vi "LINX - MMA8452Q Accelerometer.vi"() -> ()   [LabVIEW 2019]
doc: "This example demonstrates how to read X, Y, and Z accelerations using the MMA8452 accelerometer."
uses:
  <vilib>/MakerHub/LINX/Public/Utilities/Open Serial.vi
  <vilib>/MakerHub/LINX/LMH-LINX.lvlib
  <vilib>/MakerHub/LINX/Public/Sensors/Accelerometer/MMA8452/MMA8452.lvlib
panel:
  in  "Stop Button":bool
  out "Waveform Chart":T1(graph)
  in  "I2C Channel":u8
  in  "Serial Port":refnum<visa-resource-name>
  out "Loop Rate (Hz)":u32
  # "MMA8452Q Accelerometer\n\nThis example demonstrates how to read three axis of acceleration from the MMA8452Q accelerometer \n\nInstructions\n1. Select the COM Port associated with the LINX Device.\n2. Select the I2C Channel that the MMA8452Q is connected to.\n3. Click the Run Arrow."
  # "LINX Device Settings"
  # "Analog Value"
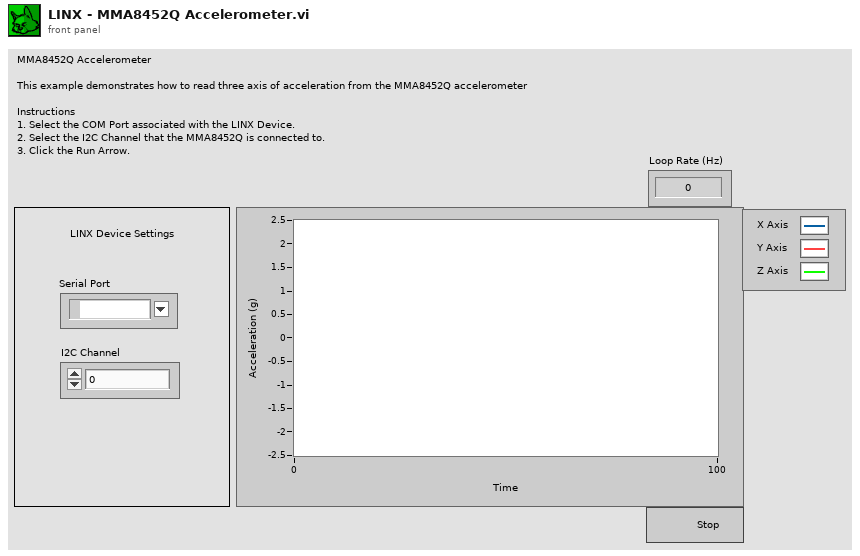
[diagram p1: front panel]
types:
  T1 = cluster{"X Axis":dbl, "Y Axis":dbl, "Z Axis":dbl}
  T2 = typedef "LMH-LINX.lvlib/LINX Ref.ctl" = cluster{"IO":T3, "Interface":T4, "LINX Device Config":T5}
  T3 = typedef "LMH-LINX.lvlib/Platform.ctl" = enum16{"Remote", "Local"}
  T4 = typedef "LMH-LINX.lvlib/Interface.ctl" = enum16{"Serial", "TCP"}
  T5 = typedef "LMH-LINX.lvlib/Device.lvlib/LINX Device Config.ctl" = cluster{"Interface":T4, "COM Port":refnum<visa-resource-name>, "TCP Configuration":T6, "Device Family":u8, "Device ID":u8, "Device Name":string, "TCP Ref":refnum<k5>, "Channels":T7}
  T6 = typedef "LMH-LINX.lvlib/Device.lvlib/TCP Config.ctl" = cluster{"IP Address":string, "Port":u16}
  T7 = typedef "LMH-LINX.lvlib/Channels.ctl" = cluster{"DI":u8[], "DO":u8[], "AI":u8[], "AO":u8[], "PWM":u8[], "QE":u8[], "UART":u8[], "I2C 2":u8[], "SPI":u8[], "CAN":u8[], "Servo":u8[], "AI Ref (V)":dbl, "AI Resolution (Bits)":u8, "AO Ref (V)":dbl, "AO Resolution (Bits)":u8}
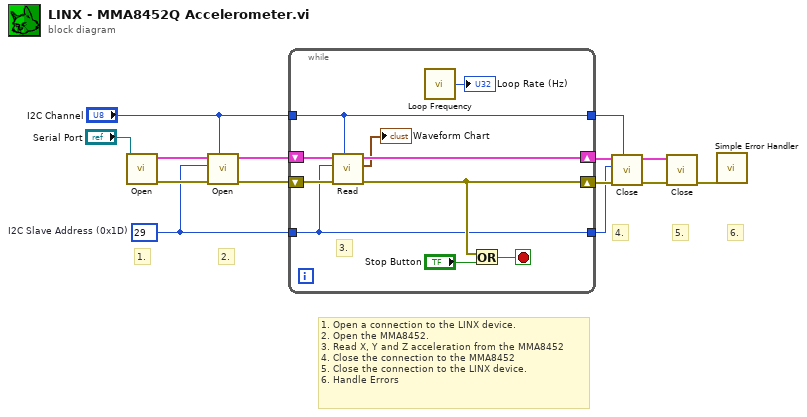
[diagram p0: block diagram]
diagram:
  w8 = u8 29  # I2C Slave Address (0x1D)
  # "6."
  # "4."
  # "2."
  # "5."
  # "1. Open a connection to the LINX device.\n2. Open the MMA8452.\n3. Read X, Y and Z acceleration from the MMA8452\n4. Close the connection to the MMA8452\n5. Close the connection to the LINX device.\n6. Handle Errors"
  # "1."
  n1 = call-poly <vilib>:"Open.vi"("Serial Port"="Serial Port") -> ("Error Out"=w13:errorcluster, "LINX Resource"=w12:T2)  [unwired: 8 in, 1 out]
  n2 = call <vilib>:"Open.vi"("I2C Channel"="I2C Channel", "Error In"=w13, "I2C Slave Address (0x1D)"=w8, "LINX Ref"=w12) -> ("Error Out"=w10:errorcluster, "LINX Resource"=w11:T2)  [unwired: 6 in]
  n3 = while {
    tunnel: "I2C Channel" -> [w17]
    tunnel: w8 -> [w15]
    shift-right: [w20] -> w5
    shift-left: w11 -> [w19]
    shift-right: [w22] -> w6
    shift-left: w10 -> [w24]
    tunnel: [w17] -> w2
    tunnel: [w15] -> w1
    stop <- w21 stop-if-true
    # "3."
    n4 = call <vilib>:"Read.vi"("I2C Channel"=w17, "Error In"=w24, "I2C Slave Address (0x1D)"=w15, "LINX Resource in"=w19) -> ("Error Out"=w22:errorcluster, "Acceleration Data (g)"=→"Waveform Chart":T1, "LINX Resource out"=w20:T2)  [unwired: 5 in]
    n5 = call <vilib>:"Loop Frequency.vi"() -> ("Loop Rate (Hz)"=→"Loop Rate (Hz)":u32)
    n6 = Or(x=w22, y="Stop Button") -> (x .or. y?=w21:bool)
  }
  n7 = call <vilib>:"Close.vi"("I2C Channel (0)"=w2, "Error In"=w6, "I2C Slave Address (0)"=w1, "LINX Resource"=w5) -> ("Error Out"=w3:errorcluster, "LINX Resource"=w4:T2)  [unwired: 6 in]
  n8 = call <vilib>:"Close.vi"("Error In"=w3, "LINX Resource"=w4) -> ("Error Out"=w7:errorcluster)  [unwired: 9 in]
  n9 = call <vilib>:"Simple Error Handler.vi"("error in (no error)"=w7) -> ()  [unwired: 4 in, 5 out]
